vi "Square Plug In.vi"(9 "Parameters":variant, 10 "Frequency":dbl, 11 "Amplitude":dbl) -> (3 "Signal out":waveform(dbl))   [LabVIEW 2011]
doc: "This is a template used in the Plug Ins exercise to simplify the process of creating a new Plug In.\n\nAAL 9/09"
uses:
  <vilib>/measure/NI_MABase.lvlib
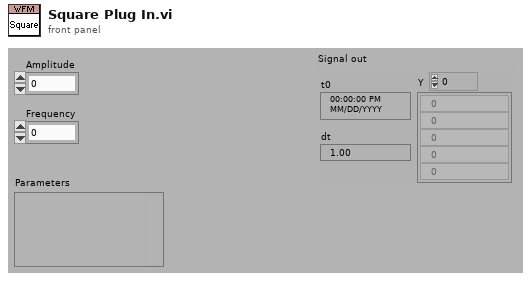
[diagram p1: front panel]
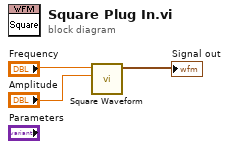
[diagram p0: block diagram]
diagram:
  n1 = call <vilib>:"Square Waveform.vi"("amplitude"="Amplitude", "frequency"="Frequency") -> ("signal out"=→"Signal out":waveform(dbl))  [unwired: 8 in, 1 out]
